vi "Create All Message Queues.vi"(8 "error in (no error)":T1 caption="entrée d'erreur (pas d'erreur)") -> (0 "error out":T1 caption="sortie d'erreur", 3 "Files d'attente de messages en sortie":T2)   [LabVIEW 2018, in "Message Queue.lvlib"]
doc: "Ce VI crée et initialise toutes les files d'attente de messages de l'application. Si votre application requiert plusieurs files d'attente de messages, cliquez sur la constante \"Message Queues\" ci-dessus avec le bouton droit et sélectionnez Ouvrir la déf. de type. Ajoutez les nouvelles files d'attente de messages à la définition de type puis initialisez-les dans ce VI."
uses:
  Message Queue.lvlib
  All Message Queues.ctl
  Message Cluster.ctl
  Enqueue Message (Single).vi
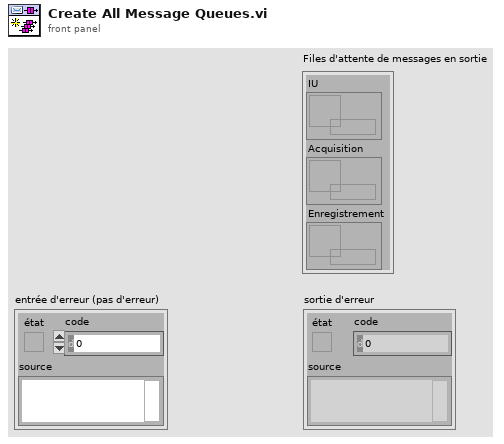
[diagram p1: front panel]
types:
  T1 = cluster{"état":bool, "code":i32, "source":string}
  T2 = typedef "Message Queue.lvlib/All Message Queues.ctl" = cluster{"IU":refnum<queue>, "Acquisition":refnum<queue>, "Enregistrement":refnum<queue>}
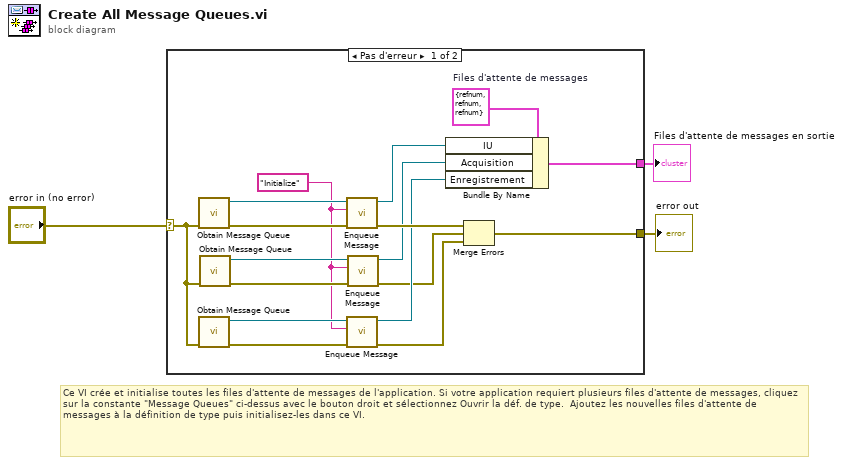
[diagram p0: block diagram]
diagram:
  # "Ce VI crée et initialise toutes les files d'attente de messages de l'application. Si votre application requiert plusieurs files d'attente de messages, cliquez sur la constante \"Message Queues\" ci-dessus avec le bouton droit et sélectionnez Ouvrir la déf. de type.  Ajoutez les nouvelles files d'attente de messages à la définition de type puis initialisez-les dans ce VI."
  n1 = case shown="Pas d'erreur" "error in (no error)" {
    selector: "error in (no error)" -> [w11 w21]
    tunnel: [w6 w21] -> w3
    tunnel: [w18 _] -> w2
    frame No Error {
      w10 = "Initialize" ("Message")
      w19 = T2 {"IU"=refnum, "Acquisition"=refnum, "Enregistrement"=refnum}  # Files d'attente de messages
      n2 = call "Obtain Message Queue.vi"("error in (no error)"=w11) -> ("error out"=w17:T1, "File d'attente de messages"=w16:refnum<queue>)  [unwired: 9 in]
      n3 = call "Obtain Message Queue.vi"("error in (no error)"=w11) -> ("error out"=w13:T1, "File d'attente de messages"=w12:refnum<queue>)  [unwired: 9 in]
      n4 = call "Obtain Message Queue.vi"("error in (no error)"=w11) -> ("error out"=w14:T1, "File d'attente de messages"=w15:refnum<queue>)  [unwired: 9 in]
      n5 = call-poly "Enqueue Message.vi"("error in (no error)"=w17, "Message"=w10, "File d'attente de messages"=w16) -> ("error out"=w20:T1, "File d'attente de message dup."=w9:refnum<queue>)  [unwired: 7 in]
      n6 = call-poly "Enqueue Message.vi"("error in (no error)"=w13, "Message"=w10, "File d'attente de messages"=w12) -> ("error out"=w4:T1, "File d'attente de message dup."=w7:refnum<queue>)  [unwired: 7 in]
      n7 = call-poly "Enqueue Message.vi"("error in (no error)"=w14, "Message"=w10, "File d'attente de messages"=w15) -> ("error out"=w5:T1, "File d'attente de message dup."=w8:refnum<queue>)  [unwired: 7 in]
      n8 = Bundle By Name(cluster=w19, "IU"=w9, "Acquisition"=w8, "Enregistrement"=w7) -> (w18:T2)
      n9 = Merge Errors(w20, w5, w4) -> (w6:errorcluster)
    }
    frame Error {
    }
  }
  "Files d'attente de messages en sortie" <- w2
  "error out" <- w3
